vi "svx_Continuous Sine Waveform.vi"(6 "sampling info":cluster{"Fs":dbl, "#s":dbl}={"Fs"=1000.0, "#s"=1000.0} {"#s" format="%.2p"; "Fs" format="%.2p"}, 7 "generation control":T2(ring), 8 "error in":errorcluster, 9 "delay until transition (0 samples)":i32, 10 "current waveform state":T3 {"tf" format="%.2f"; "offset" format="%.2f"; "phase in" format="%.2f"; "amplitude" format="%.2f"; "frequency" format="%.2f"}, 11 "desired waveform state":T1={"frequency"=10.0, "amplitude"=1.0, "phase"=0.0, "offset"=0.0, "tf (ignored)"=0.0} {"tf (ignored)" format="%.2f"; "phase" format="%.2f"; "offset" format="%.2p"; "amplitude" format="%.2p"; "frequency" format="%.2p"}) -> (0 "error out":errorcluster, 1 "index of transition":i32, 2 "next waveform state":T3 {"tf" format="%.2f"; "offset" format="%.2f"; "phase in" format="%.2f"; "amplitude" format="%.2f"; "frequency" format="%.2f"}, 3 "signal out":waveform(dbl))   [LabVIEW 2017]
doc: "Continuous Sine Waveform generates a waveform containing a sine wave. If the frequency or amplitude of the sine wave changes, the VI changes the state of the sine wave at the next available zero crossing."
uses:
  <vilib>/Analysis/NI_AALBase.lvlib
  <vilib>/measure/NI_MABase.lvlib
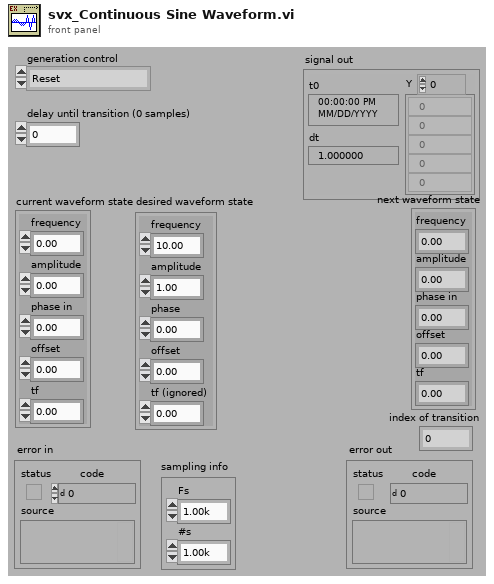
[diagram p1: front panel]
types:
  T1 = cluster{"frequency":dbl, "amplitude":dbl, "phase":dbl, "offset":dbl, "tf (ignored)":dbl}
  T2 = enum16{"Reset", "Continue from previous", "Continue from state", "Zero from previous", "Zero from state"}
  T3 = cluster{"frequency":dbl, "amplitude":dbl, "phase in":dbl, "offset":dbl, "tf":dbl}
  T4 = cluster{"frequency":dbl, "amplitude":dbl, "phase out":dbl, "offset":dbl, "tf new":dbl}
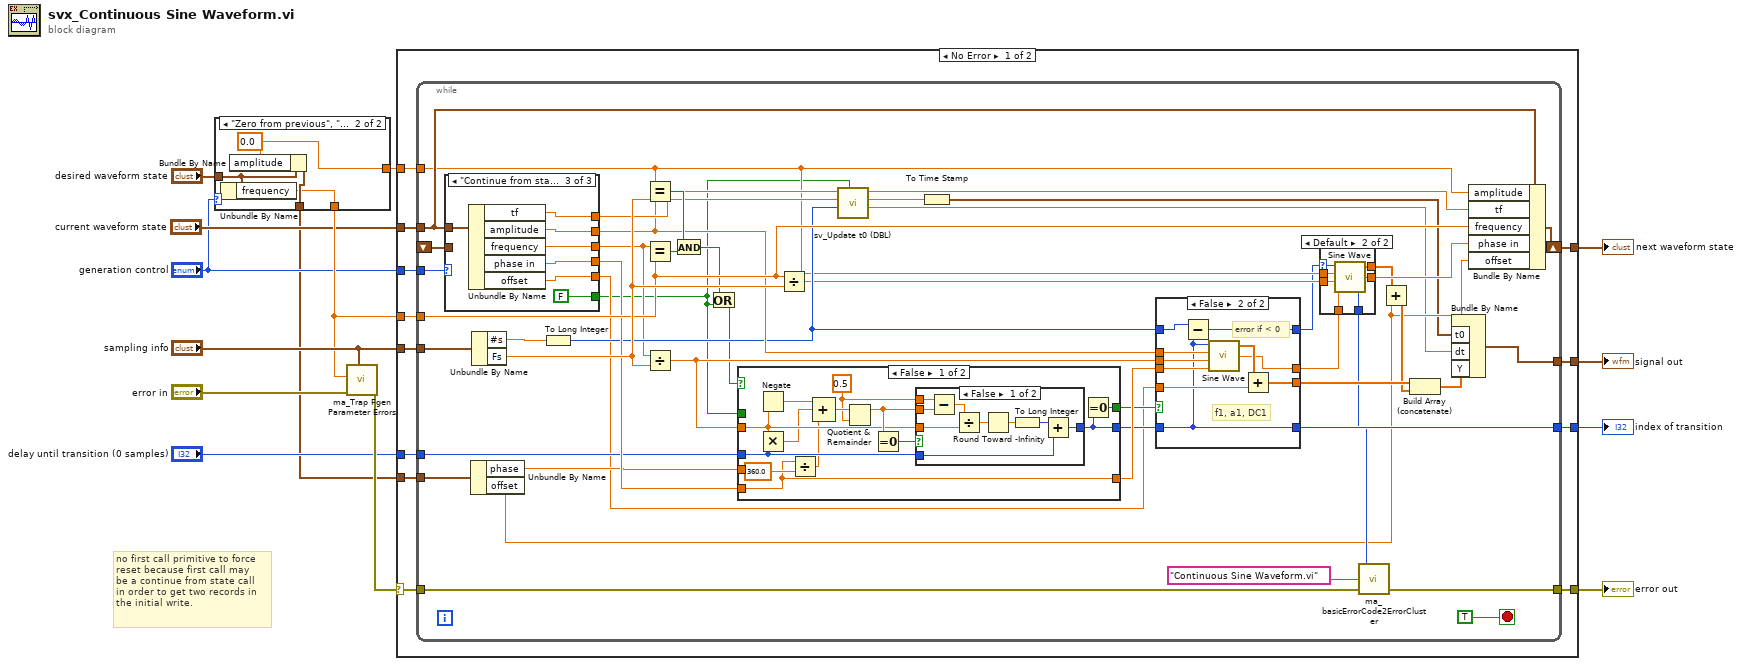
[diagram p0: block diagram]
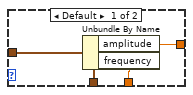
[diagram p2: hidden frame]
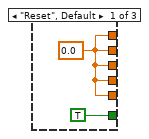
[diagram p4: hidden frame]
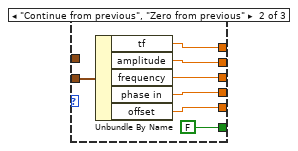
[diagram p5: hidden frame]
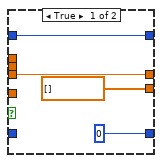
[diagram p6: hidden frame]
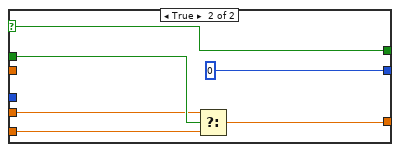
[diagram p8: hidden frame]
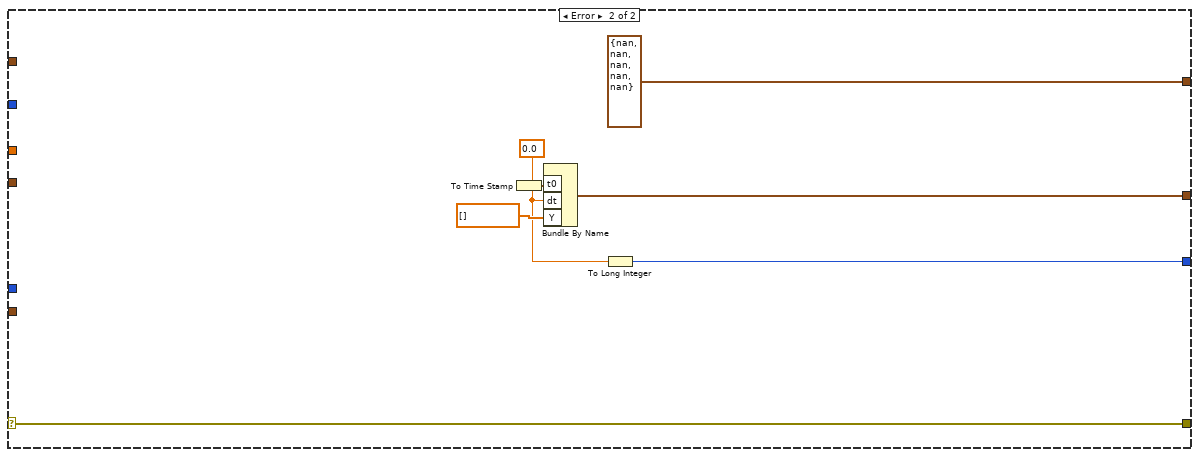
[diagram p9: hidden frame]
diagram:
  # "no first call primitive to force \nreset because first call may \nbe a continue from state call\nin order to get two records in \nthe initial write."
  n1 = case shown="\"Zero from previous\", \"Zero from state\"" "generation control" {
    tunnel: [w17 w20] -> w7
    tunnel: [w15 w18] -> w6
    tunnel: "desired waveform state" -> [w16 w19]
    tunnel: [w16 w21] -> w2
    frame Default {
      n2 = Unbundle By Name(w16) -> ("amplitude"=w17:dbl, "frequency"=w15:dbl)
    }
    frame "Zero from previous", "Zero from state" {
      w20 = 0.0 ("amplitude")
      n3 = Unbundle By Name(w19) -> ("frequency"=w18:dbl)
      n4 = Bundle By Name(cluster=w19, "amplitude"=w20) -> (w21:T1)
    }
  }
  n5 = call <vilib>:"ma_Trap Fgen Parameter Errors.vi"("Sampling info"="sampling info", "error in (no error)"="error in", "frequency"=w6) -> ("error out"=w11:errorcluster)  [unwired: 8 in]
  n6 = case shown="No Error" w11 {
    selector: w11 -> [w30 w153]
    tunnel: "sampling info" -> [w33 _]
    tunnel: w6 -> [w28 _]
    tunnel: [w32 w153] -> w13
    tunnel: [w31 w154] -> w1
    tunnel: w7 -> [w29 _]
    tunnel: [w27 w150] -> w10
    tunnel: "delay until transition (0 samples)" -> [w26 _]
    tunnel: [w25 T4 {"frequency"=nan, "amplitude"=nan, "phase out"=nan, "offset"=nan, "tf new"=nan}] -> w8
    tunnel: "generation control" -> [w24 _]
    tunnel: w2 -> [w23 _]
    tunnel: "current waveform state" -> [w22 _]
    frame No Error {
      n7 = while {
        tunnel: w22 -> [w45]
        tunnel: w23 -> [w54]
        tunnel: w24 -> [w61]
        shift-left: _ -> [w60]
        shift-right: [w38] -> w25
        tunnel: w26 -> [w51]
        tunnel: [w73] -> w27
        tunnel: w28 -> [w63]
        tunnel: w29 -> [w42]
        tunnel: w30 -> [w76]
        tunnel: [w77] -> w31
        tunnel: [w78] -> w32
        tunnel: w33 -> [w79]
        stop <- TRUE stop-if-true
        n8 = case shown="\"Continue from state\", \"Zero from state\"" w61 {
          tunnel: w60 -> [_ w96 _]
          tunnel: [TRUE FALSE FALSE] -> w36
          tunnel: [w89 w91 w99] -> w59
          tunnel: [w89 w95 w101] -> w58
          tunnel: [w89 w94 w103] -> w49
          tunnel: [w89 w93 w100] -> w57
          tunnel: [w89 w92 w102] -> w41
          tunnel: w45 -> [_ _ w98]
          frame "Reset", Default {
            w89 = 0.0
          }
          frame "Continue from previous", "Zero from previous" {
            n9 = Unbundle By Name(w96) -> ("tf"=w91:dbl, "amplitude"=w95:dbl, "frequency"=w94:dbl, "phase in"=w93:dbl, "offset"=w92:dbl)
          }
          frame "Continue from state", "Zero from state" {
            n10 = Unbundle By Name(w98) -> ("tf"=w99:dbl, "amplitude"=w101:dbl, "frequency"=w103:dbl, "phase in"=w100:dbl, "offset"=w102:dbl)
          }
        }
        n11 = Unbundle By Name(w54) -> ("phase"=w53:dbl, "offset"=w39:dbl)
        n12 = Unbundle By Name(w79) -> ("#s"=w52:dbl, "Fs"=w70:dbl)
        n13 = To Long Integer(number=w52) -> (32bit integer=w55:i32)
        n14 = Equal?(x=w42, y=w58) -> (x = y?=w75:bool)
        n15 = Equal?(x=w49, y=w63) -> (x = y?=w74:bool)
        n16 = Divide(x=w49, y=w70) -> (x/y=w69:dbl)
        n17 = And(x=w75, y=w74) -> (x .and. y?=w47:bool)
        n18 = Or(x=w47, y=w36) -> (x .or. y?=w46:bool)
        n19 = case shown="False" w46 {
          selector: w46 -> [_ w147]
          tunnel: [w119 w142] -> w68
          tunnel: w57 -> [w119 w143]
          tunnel: w69 -> [w124 _]
          tunnel: w51 -> [w125 _]
          tunnel: w53 -> [_ w144]
          tunnel: [w130 w147] -> w48
          tunnel: [w128 0] -> w50
          tunnel: w36 -> [_ w145]
          frame False {
            w129 = 0.5 ("y")
            n20 = Negate(x=w124) -> (-x=w123:dbl)
            n21 = Multiply(x=w124, y=w125) -> (x*y=w122:dbl)
            n22 = Divide(x=w119, y=360.0) -> (x/y=w121:dbl)
            n23 = Compound Arithmetic op=ADD(w123, w122, w121) -> (w131:dbl)
            n24 = Quotient & Remainder(x=w131, y=w129) -> (x-y*floor(x/y)=w127:dbl)  [unwired: 1 out]
            n25 = Equal To 0?(x=w127) -> (x = 0?=w126:bool)
            n26 = case shown="False" w126 {
              tunnel: w124 -> [w137 _]
              tunnel: w127 -> [w136 _]
              tunnel: w129 -> [w135 _]
              tunnel: w125 -> [w133 w141]
              tunnel: [w134 w141] -> w128
              frame False {
                n27 = Subtract(x=w135, y=w136) -> (x-y=w138:dbl)
                n28 = Divide(x=w138, y=w137) -> (x/y=w139:dbl)
                n29 = Round Toward -Infinity(1:w139) -> (0:w132:dbl)
                n30 = To Long Integer(number=w132) -> (32bit integer=w140:i32)
                n31 = Add(x=w140, y=w133) -> (x+y=w134:i32)
              }
              frame True {
              }
            }
            n32 = Equal To 0?(x=w128) -> (x = 0?=w130:bool)
          }
          frame True {
            n33 = Select(t=w144, s=w145, f=w143) -> (s? t:f=w142:dbl)
          }
        }
        n34 = Divide(x=w63, y=w70) -> (x/y=w44:dbl)
        n35 = call <vilib>:"sv_Update t0 (DBL).vi"("Reset Generation"=w36, "samples"=w55, "sample rate (S/s)"=w70, "tf previous"=w59) -> ("dt"=w35:dbl, "t0"=w56:dbl, "tf new"=w64:dbl)  [unwired: 5 in]
        n36 = To Time Stamp(1:w56) -> (0:w34:timestamp)
        n37 = case shown="False" w48 {
          tunnel: [w106 w109] -> w43
          tunnel: w68 -> [w106 w112]
          tunnel: w55 -> [w105 w113]
          tunnel: w58 -> [_ w118]
          tunnel: [0 w111] -> w73
          tunnel: [dbl[] [] ("Sine Wave") w115] -> w72
          tunnel: [w105 w117] -> w37
          tunnel: w69 -> [_ w116]
          tunnel: w41 -> [_ w114]
          tunnel: w50 -> [_ w111]
          frame True {
          }
          frame False {
            # "error if < 0"
            # "f1, a1, DC1"
            n38 = Subtract(x=w113, y=w111) -> (x-y=w117:i32)
            n39 = call <vilib>:"Sine Wave.vi"("samples"=w111, "amplitude"=w118, "frequency"=w116, "phase in"=w112) -> ("sine wave"=w110:dbl[], "phase out"=w109:dbl)  [unwired: 1 in, 1 out]
            n40 = Add(x=w110, y=w114) -> (x+y=w115:dbl[])
          }
        }
        n41 = case shown="Default" w37 {
          selector: w37 -> [_ w82]
          tunnel: [_ w88] -> w71
          tunnel: [w81 w87] -> w62
          tunnel: w44 -> [_ w86]
          tunnel: w43 -> [w81 w85]
          tunnel: w42 -> [_ w84]
          tunnel: [_ w83] -> w40
          frame 0 {
          }
          frame Default {
            n42 = call <vilib>:"Sine Wave.vi"("samples"=w82, "amplitude"=w84, "frequency"=w86, "phase in"=w85) -> ("sine wave"=w83:dbl[], "phase out"=w87:dbl, "error"=w88:i32)  [unwired: 1 in]
          }
        }
        n43 = call <vilib>:"ma_basicErrorCode2ErrorCluster.vi"("error in (no error)"=w76, "subVI name"="Continuous Sine Waveform.vi" ("subVI Name"), "Error Code"=w71) -> ("error out"=w78:errorcluster)
        n44 = Add(x=w40, y=w39) -> (x+y=w67:dbl[])
        n45 = Build Array (concatenate)(w72, w67) -> (w66:dbl[])
        n46 = Bundle By Name("t0"=w34, "dt"=w35, "Y"=w66) -> (w77:waveform(dbl))  [unwired: 1 in]
        n47 = Bundle By Name(cluster=w45, "amplitude"=w42, "tf"=w64, "frequency"=w63, "phase in"=w62, "offset"=w39) -> (w38:T3)
      }
    }
    frame Error {
      w151 = 0.0 ("t0")
      n48 = To Time Stamp(1:w151) -> (0:w148:timestamp)
      n49 = Bundle By Name("t0"=w148, "dt"=w151, "Y"=dbl[] []) -> (w154:waveform(dbl))  [unwired: 1 in]
      n50 = To Long Integer(number=w151) -> (32bit integer=w150:i32)
    }
  }
  "error out" <- w13
  "signal out" <- w1
  "index of transition" <- w10
  "next waveform state" <- w8
